vi "Teleop.vi"(10 "Match Info":T1={"Autonomous Elapsed Seconds"=0.0, "TeleOp Elapsed Seconds"=0.0, "Disabled Elapsed Seconds"=0.0, "Visited Autonomous"=FALSE, "Visited TeleOp"=FALSE, "Visited Disabled"=FALSE, "Autonomous Settings"={"Autonomous Style"=enum."Independent", "VI Refnum"=refnum}}, 11 "Call Context":T2) -> ()   [LabVIEW 2015]
doc: "This VI is called for each TeleOp packet received from the DS where the robot is not disabled. It is often used to read from the joysticks and update I/O or to update setpoints for timed control loops. It should complete and return within 20 milliseconds or it may miss DS packets."
uses:
  <vilib>/Rock Robotics/WPI/DriverStation/WPI_DriverStationDerivedRobotMode.ctl
  <vilib>/Rock Robotics/WPI/DriverStation/WPI_DriverStationMatch Info.ctl
  <vilib>/Rock Robotics/WPI/Utilities/WPI_GetSetVariantRefNum.vi
  Robot Global Data.vi
  <vilib>/Rock Robotics/Network Tables/SD Write Number.vi
  <vilib>/Rock Robotics/WPI/Solenoid/Deprecated/WPI_SolenoidSetBool.vi
  <vilib>/Rock Robotics/Network Tables/NT Write Number.vi
  <vilib>/Rock Robotics/Network Tables/NT Write Boolean.vi
  Z navX/navX Library v2/navX Library v2.lvlib
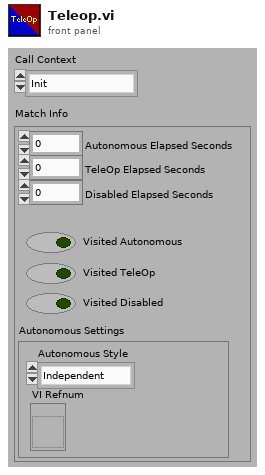
[diagram p1: front panel]
types:
  T1 = typedef "WPI_DriverStationMatch Info.ctl" = cluster{"Autonomous Elapsed Seconds":dbl, "TeleOp Elapsed Seconds":dbl, "Disabled Elapsed Seconds":dbl, "Visited Autonomous":bool, "Visited TeleOp":bool, "Visited Disabled":bool, "Autonomous Settings":cluster{"Autonomous Style":enum16{"Iterative", "Independent"}, "VI Refnum":refnum<vi>}}
  T2 = typedef "WPI_DriverStationDerivedRobotMode.ctl" = enum16{"Init", "Execute", "Stop"}
  T3 = enum16{"No Override", "Override to Coast", "Override to Brake"}
  T4 = typedef "WPI_JoystickDevRef.ctl" = cluster{"Device":T5}
  T5 = typedef "WPI_JoystickDeviceEnum.ctl" = enum16{"USB 0", "USB 1", "USB 2", "USB 3", "USB 4", "USB 5"}
  T6 = cluster{"Axes[0]":dbl, "Axes[1]":dbl, "Axes[2]":dbl, "Axes[3]":dbl, "Axes[4]":dbl, "Axes[5]":dbl, "Axes[6]":dbl, "Axes[7]":dbl, "Axes[8]":dbl}
  T7 = cluster{"Buttons[0]":bool, "Buttons[1]":bool, "Buttons[2]":bool, "Buttons[3]":bool, "Buttons[4]":bool, "Buttons[5]":bool, "Buttons[6]":bool, "Buttons[7]":bool, "Buttons[8]":bool}
  T8 = typedef "navX Library v2.lvlib/Z900_navX_DeviceTypeDef.ctl" = cluster{"Interface":cluster{"Protocol":T9, "Update Rate (4Hz-60Hz)":u8, "navX Open TypeDef":variant}, "Notify Packet":refnum<notifier>, "Loop VI Refnum":refnum<vi>, "Ready to Close Occurrence Refnum":refnum<k4>}
  T9 = typedef "navX Library v2.lvlib/Z900_navX_ProtocolTypeDef.ctl" = enum16{"SERIAL", "I2C", "SPI"}
  T10 = cluster{"Yaw":dbl, "Roll":dbl, "Pitch":dbl, "Heading":dbl, "Fused Heading":dbl}
  T11 = cluster{"LinearAcceleration X":dbl, "LinearAcceleration Y":dbl, "LinearAcceleration Z":dbl}
  T12 = cluster{"Velocity X":dbl, "Velocity Y":dbl, "Velocity Z":dbl, "Displacement X":dbl, "Displacement Y":dbl, "Displacement Z":dbl}
  T13 = typedef "WPI_MotorControlDeviceRef.ctl" = cluster{"DeviceStatus":errorcluster, "Type":T14, "PWM":cluster{"PWM Channel":T15, "DeadBand":T16}, "CAN":cluster{"Device Number":u8, "Control Mode":T17, "Semaphore":T18, "Max Vout":dbl, "TalonSRX Control Mode":T19}, "Invert":bool}
  T14 = typedef "WPI_MotorControlType.ctl" = enum16{"PWM", "CAN", "CANTalonSRX"}
  T15 = typedef "FPGA_DIOPWMChannel.ctl" = enum8{"PWM 0", "PWM 1", "PWM 2", "PWM 3", "PWM 4", "PWM 5", "PWM 6", "PWM 7", "PWM 8", "PWM 9", "PWM MXP 0", "PWM MXP 1", "PWM MXP 2", "PWM MXP 3", "PWM MXP 4", "PWM MXP 5", "PWM MXP 6", "PWM MXP 7", "PWM MXP 8", "PWM MXP 9", "Invalid"}
  T16 = typedef "WPI_PWMDeadband.ctl" = cluster{"Name":string, "maxPositivePwm":i32, "minPositivePwm":i32, "centerPwm":i32, "maxNegativePwm":i32, "minNegativePwm":i32, "angularRange":u16}
  T17 = typedef "WPI_CANJaguar_ControlMode.ctl" = enum8{"Percent VBus", "Current", "Speed", "Position", "Voltage"}
  T18 = typedef "Semaphore RefNum" = refnum<k1>
  T19 = typedef "WPI_CANTalonSRX_APIControlMode.ctl" = enum8{"Percent VBus", "Speed", "Position", "Slave", "Unchanged / Invalid", "Voltage Compensation", "Current", "Motion Profile"}
  T20 = typedef "WPI_SolenoidDevRef.ctl" = cluster{"DevStatus":errorcluster, "Pneumatics Control Module":u8, "Forward Solenoid Channel":T21, "Reverse Solenoid Channel":T21}
  T21 = typedef "WPI_SolenoidChannel.ctl" = enum8{"Solenoid 0", "Solenoid 1", "Solenoid 2", "Solenoid 3", "Solenoid 4", "Solenoid 5", "Solenoid 6", "Solenoid 7", "Invalid"}
  T22 = typedef "WPI_CANTalonSRX_GlobalStatus.ctl" = cluster{"Applied Throttle":dbl, "Module Enabled":bool, "CAN Error":errorcluster, "Closed Loop Error":dbl, "Forward Limit Switch Closed":bool, "Reverse Limit Switch Closed":bool, "Sensor Position":dbl, "Sensor Velocity":dbl, "Current":dbl, "Sticky Fault - Over Temp":bool, "Sticky Fault - Under Voltage":bool, "Sticky Fault - Forward Limit":bool, "Sticky Fault - Reverse Limit":bool, "Sticky Fault - Forward Soft Limit":bool, "Sticky Fault - Reverse Soft Limit":bool, "Brake is Enabled":bool, "Encoder Position":dbl, "Encoder Velocity":dbl, "Encoder Index Count":dbl, "Encoder A Pin State":bool, "Encoder B Pin State":bool, "Encoder Index Pin State":bool, "Analog In":dbl, "Analog In Velocity":dbl, "Temperature (C)":dbl, "Battery Voltage":dbl, "Control 5 Is Supported":bool, "Current Profile Slot Select":dbl, "Pos Div 8":bool, "Vel Div 4":bool, "Pulse Width Position":i32, "Pulse Width Velocity":i32, "Pulse Width Rise To Rise (us)":i32, "Pulse Width Rise To Fall (us)":i32, "Mot Prof Active Is Under Run":bool, "Mot Prof Active Has Under Run":bool, "Mot Prof Active Is Last":bool, "Mot Prof Active Velocity Only":bool, "Mot Prof Active Is Valid":bool, "Mot Prof Buffer Is Full":bool, "Mot Prof Active Profile Slot Select":i32, "Mot Prof NextID":i32, "Mot Prof Count":i32, "Mot Prof Active Velocity":dbl, "Mot Prof Active Position":dbl, "Mot Prof Output Enable":i32}
  T23 = typedef "WPI_RobotDriveDevRef.ctl" = cluster{"DevStatus":errorcluster, "Motors[]":T13[], "Square Inputs":bool, "Max Output":dbl}
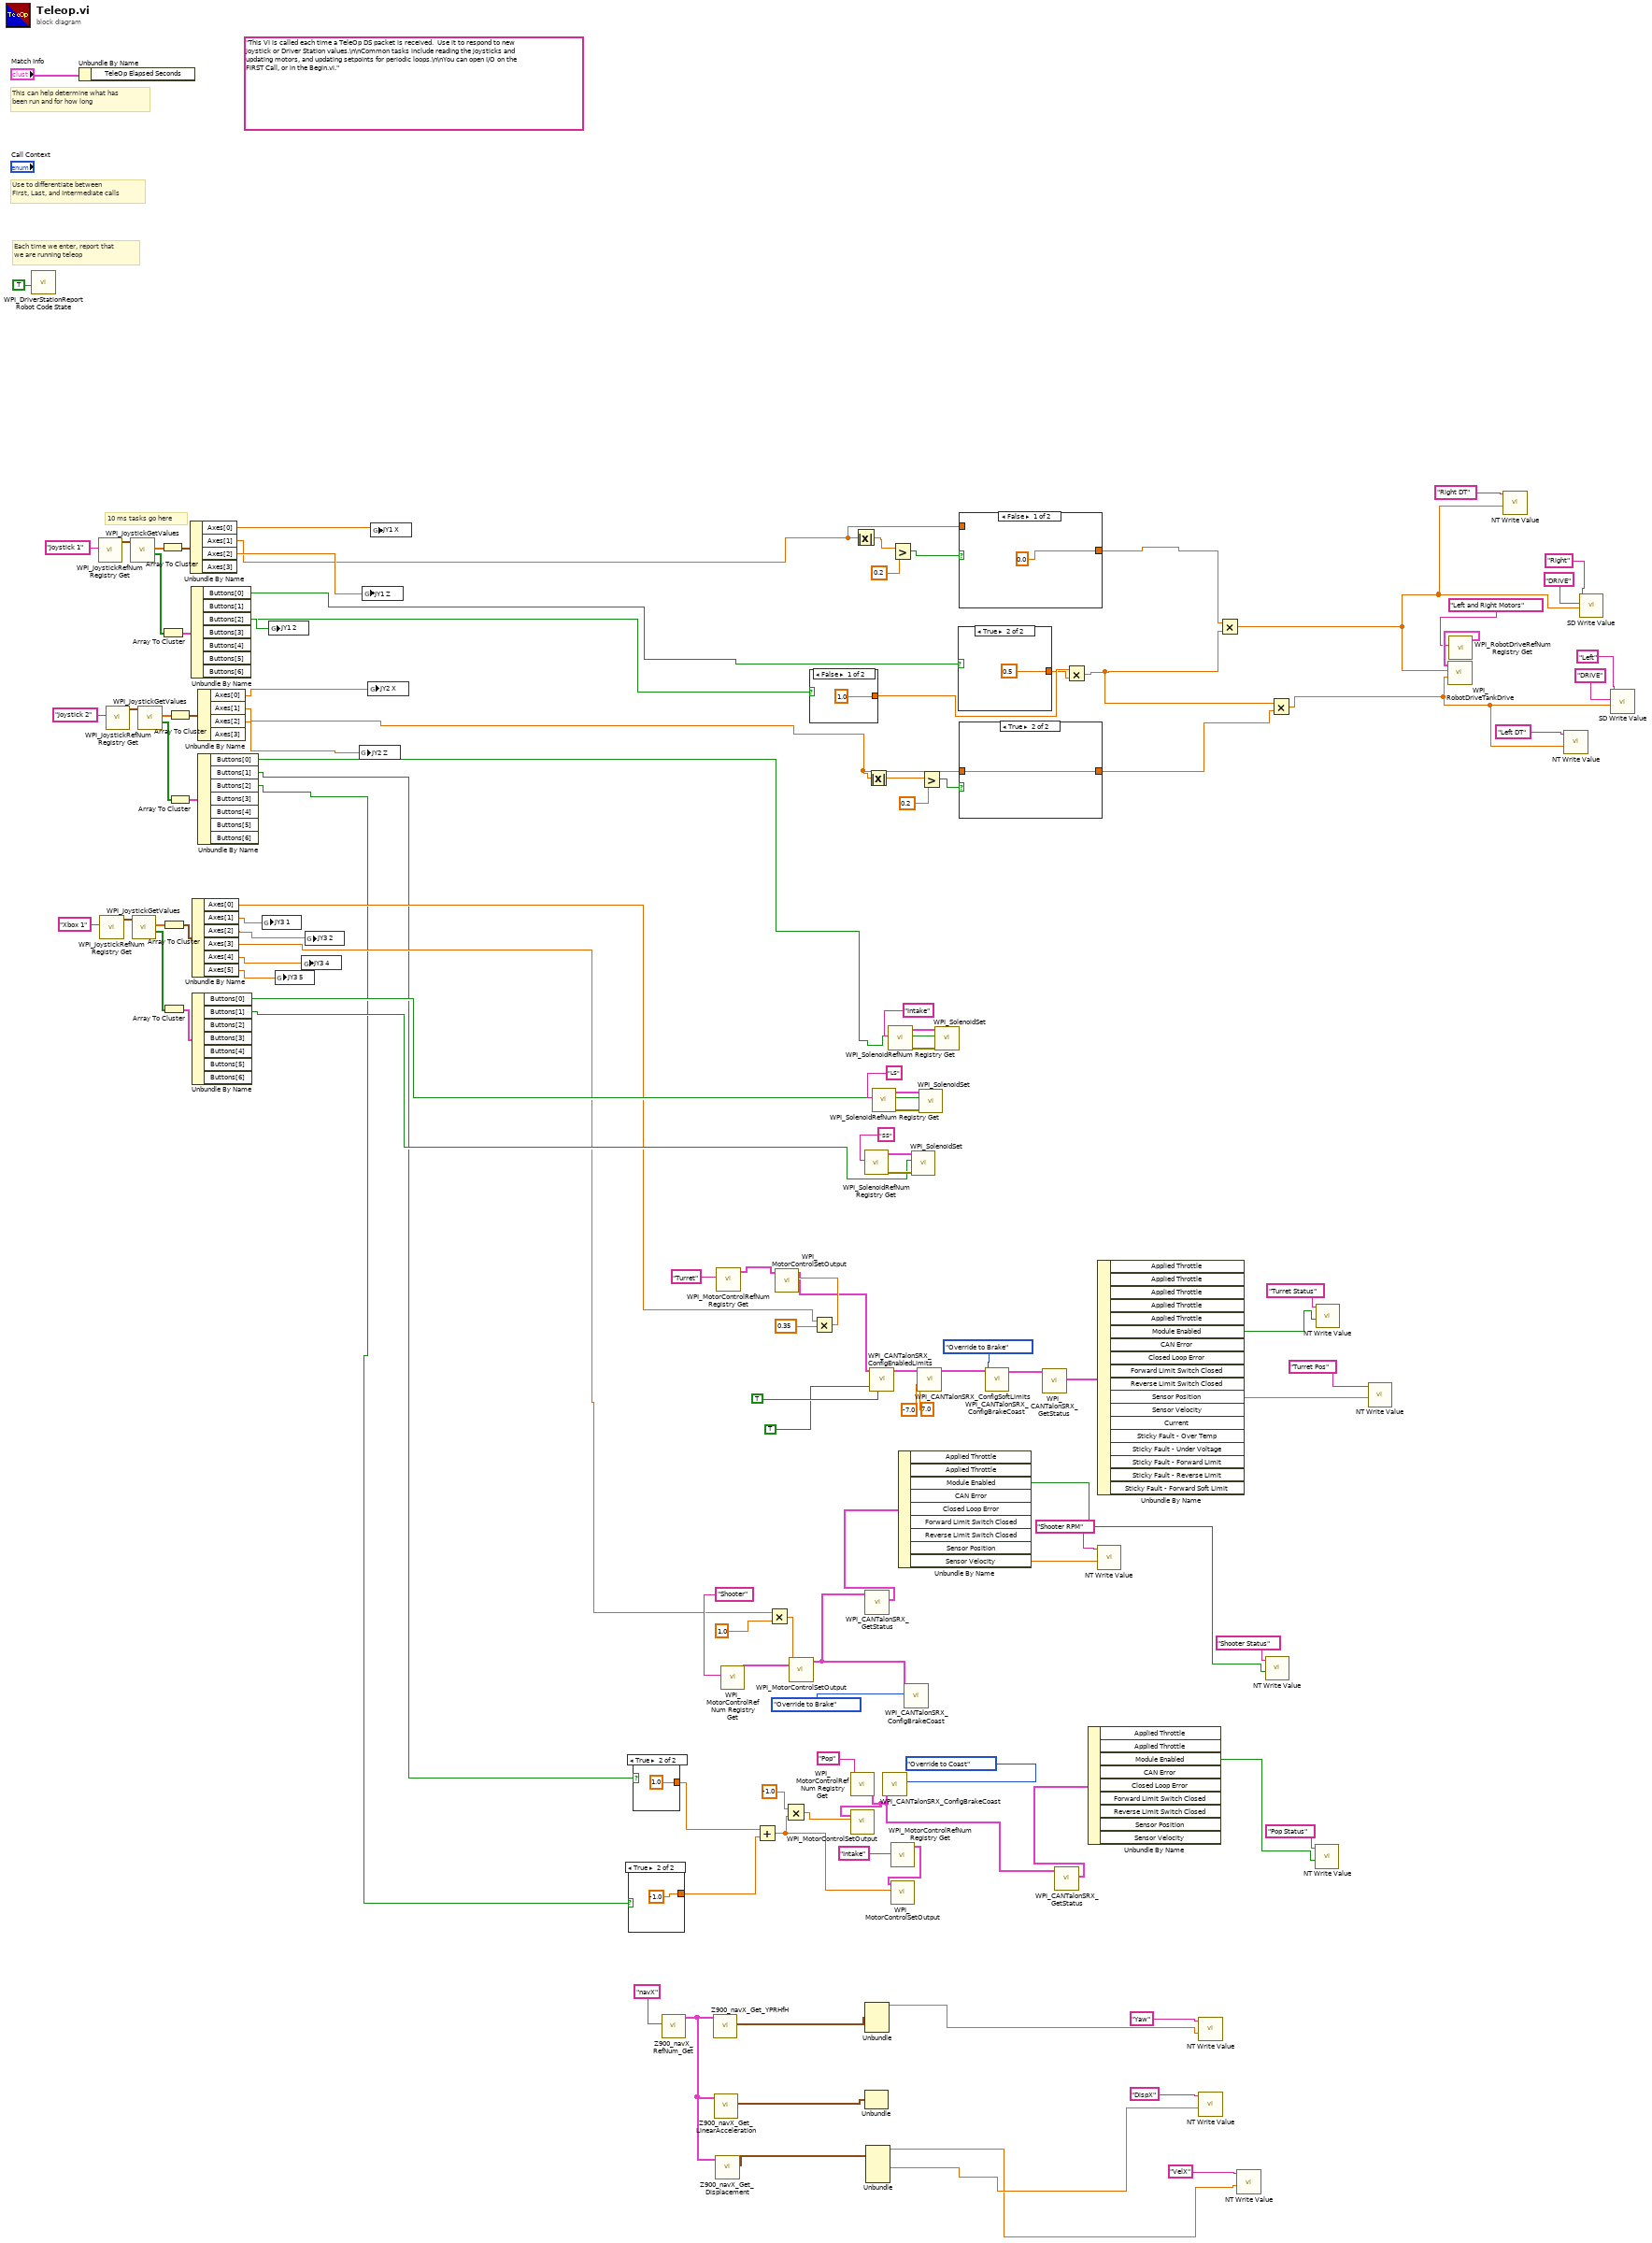
[diagram p0: block diagram]
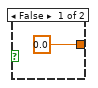
[diagram p2: hidden frame]
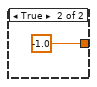
[diagram p3: hidden frame]
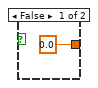
[diagram p4: hidden frame]
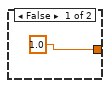
[diagram p5: hidden frame]
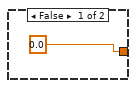
[diagram p6: hidden frame]
diagram:
  (unwired) "This VI is called each time a TeleOp DS packet is received.  Use it to respond to new joystick or Driver Station values.\n\nCommon tasks include reading the joysticks and updating motors, and updating setpoints for periodic loops.\n\nYou can open I/O on the FIRST Call, or in the Begin.vi."
  # "10 ms tasks go here"
  # "Each time we enter, report that\nwe are running teleop"
  # "Use to differentiate between\nFirst, Last, and Intermediate calls"
  # "This can help determine what has\nbeen run and for how long"
  n1 = call <vilib>:"WPI_DriverStationReport Robot Code State.vi"("TeleOp"=TRUE ("Autonomous")) -> ()  [unwired: 10 in, 1 out]
  n2 = Unbundle By Name("Match Info") -> ()  [unwired: 1 out]
  n3 = call <vilib>:"WPI_JoystickRefNum Registry Get.vi"("refnum name"="Joystick 1") -> ("JoystickDevRef"=w77:T4)  [unwired: 1 in, 9 out]
  n4 = call <vilib>:"WPI_JoystickRefNum Registry Get.vi"("refnum name"="Xbox 1") -> ("JoystickDevRef"=w65:T4)  [unwired: 1 in, 9 out]
  n5 = call <vilib>:"WPI_JoystickRefNum Registry Get.vi"("refnum name"="Joystick 2") -> ("JoystickDevRef"=w71:T4)  [unwired: 1 in, 9 out]
  n6 = call <vilib>:"WPI_JoystickGetValues.vi"("JoystickDevRef"=w77) -> ("Buttons"=w75:bool[], "Axes"=w74:dbl[])  [unwired: 6 in, 3 out]
  n7 = call <vilib>:"WPI_JoystickGetValues.vi"("JoystickDevRef"=w65) -> ("Buttons"=w63:bool[], "Axes"=w62:dbl[])  [unwired: 6 in, 3 out]
  n8 = call <vilib>:"WPI_JoystickGetValues.vi"("JoystickDevRef"=w71) -> ("Buttons"=w69:bool[], "Axes"=w68:dbl[])  [unwired: 6 in, 3 out]
  n9 = Array To Cluster(array=w74) -> (cluster=w76:T6)
  n10 = Array To Cluster(array=w75) -> (cluster=w73:T7)
  n11 = Array To Cluster(array=w62) -> (cluster=w64:T6)
  n12 = Array To Cluster(array=w63) -> (cluster=w61:T7)
  n13 = Array To Cluster(array=w68) -> (cluster=w70:T6)
  n14 = Array To Cluster(array=w69) -> (cluster=w67:T7)
  n15 = Unbundle By Name(w76) -> ("Axes[0]"=w59:dbl, "Axes[1]"=w49:dbl, "Axes[2]"=w58:dbl)  [unwired: 1 out]
  n16 = Unbundle By Name(w73) -> ("Buttons[0]"=w51:bool, "Buttons[1]"=w50:bool, "Buttons[2]"=w52:bool)  [unwired: 4 out]
  n17 = Unbundle By Name(w64) -> ("Axes[0]"=w31:dbl, "Axes[1]"=w55:dbl, "Axes[2]"=w53:dbl, "Axes[3]"=w40:dbl, "Axes[4]"=w54:dbl, "Axes[5]"=w60:dbl)
  n18 = Unbundle By Name(w61) -> ("Buttons[0]"=w46:bool, "Buttons[1]"=w45:bool)  [unwired: 5 out]
  n19 = Unbundle By Name(w70) -> ("Axes[0]"=w57:dbl, "Axes[1]"=w48:dbl, "Axes[2]"=w56:dbl)  [unwired: 1 out]
  n20 = Unbundle By Name(w67) -> ("Buttons[0]"=w47:bool, "Buttons[1]"=w24:bool, "Buttons[2]"=w23:bool)  [unwired: 4 out]
  n21 = global write "Robot Global Data.vi" "JY3 1"(w55) -> ()
  n22 = global write "Robot Global Data.vi" "JY1 2"(w52) -> ()
  n23 = global write "Robot Global Data.vi" "JY3 5"(w60) -> ()
  n24 = global write "Robot Global Data.vi" "JY3 4"(w54) -> ()
  n25 = global write "Robot Global Data.vi" "JY3 2"(w53) -> ()
  n26 = global write "Robot Global Data.vi" "JY2 Z"(w56) -> ()
  n27 = global write "Robot Global Data.vi" "JY1 Z"(w58) -> ()
  n28 = global write "Robot Global Data.vi" "JY2 X"(w57) -> ()
  n29 = global write "Robot Global Data.vi" "JY1 X"(w59) -> ()
  n30 = case shown="True" w23 {
    tunnel: [0.0 -1.0] -> w90
    frame False {
    }
    frame True {
    }
  }
  n31 = case shown="True" w24 {
    tunnel: [0.0 1.0] -> w91
    frame False {
    }
    frame True {
    }
  }
  n32 = call "Z900_navX_RefNum_Get.vi"("refnum name"="navX") -> ("navX Device"=w43:T8)  [unwired: 9 in, 1 out]
  n33 = call "Z900_navX_Get_YPRHfH.vi"("navX Device"=w43) -> ("YRPHfH"=w44:T10)  [unwired: 7 in, 3 out]
  n34 = call "Z900_navX_Get_LinearAcceleration.vi"("navX Device"=w43) -> ("Linear Acceleration"=w42:T11)  [unwired: 7 in, 3 out]
  n35 = call "Z900_navX_Get_Displacement.vi"("navX Device"=w43) -> ("Displacement"=w41:T12)  [unwired: 7 in, 3 out]
  n36 = call <vilib>:"WPI_MotorControlRefNum Registry Get.vi"("refnum name"="Turret") -> ("MotorControlDevRef"=w30:T13)  [unwired: 9 in, 1 out]
  n37 = call <vilib>:"WPI_MotorControlRefNum Registry Get.vi"("refnum name"="Shooter") -> ("MotorControlDevRef"=w86:T13)  [unwired: 9 in, 1 out]
  n38 = Add(x=w91, y=w90) -> (x+y=w84:dbl)
  n39 = Multiply(x=w40, y=1.0) -> (x*y=w89:dbl)
  n40 = Multiply(x=-1.0, y=w84) -> (x*y=w85:dbl)
  n41 = call <vilib>:"WPI_MotorControlSetOutput.vi"("Output"=w89, "MotorControlDevRef"=w86) -> ("MotorControlDevRef"=w81:T13)  [unwired: 7 in, 2 out]
  n42 = case shown="False" w50 {
    tunnel: [1.0 -1.0] -> w96
    frame False {
    }
    frame True {
    }
  }
  n43 = Multiply(x=w31, y=0.35) -> (x*y=w38:dbl)
  n44 = call <vilib>:"WPI_MotorControlSetOutput.vi"("Output"=w38, "MotorControlDevRef"=w30) -> ("MotorControlDevRef"=w29:T13)  [unwired: 7 in, 2 out]
  n45 = call <vilib>:"WPI_MotorControlRefNum Registry Get.vi"("refnum name"="Pop") -> ("MotorControlDevRef"=w3:T13)  [unwired: 9 in, 1 out]
  n46 = call <vilib>:"WPI_MotorControlSetOutput.vi"("Output"=w85, "MotorControlDevRef"=w3) -> ()  [unwired: 7 in, 3 out]
  n47 = Absolute Value(x=w49) -> (abs(x)=w117:dbl)
  n48 = call <vilib>:"WPI_SolenoidRefNum Registry Get.vi"("refnum name"="SS") -> ("error out"=w103:errorcluster, "SolenoidDevRef"=w104:T20)  [unwired: 9 in]
  n49 = Unbundle(w42) -> ()  [unwired: 3 out]
  n50 = call <vilib>:"WPI_CANTalonSRX_GetStatus.vi"("CAN Talon SRX Ref"=w81) -> ("Talon SRX Status"=w87:T22)  [unwired: 8 in, 2 out]
  n51 = Unbundle(w44) -> ("Yaw"=w10:dbl)  [unwired: 4 out]
  n52 = Unbundle(w41) -> ("Velocity X"=w8:dbl, "Displacement X"=w12:dbl)  [unwired: 4 out]
  n53 = Absolute Value(x=w48) -> (abs(x)=w116:dbl)
  n54 = call <vilib>:"WPI_CANTalonSRX_ConfigEnabledLimits.vi"("CAN Talon SRX Ref"=w29, "Forward Soft Limit Enable"=TRUE, "Reverse Soft Limit Enable"=TRUE) -> ("CAN Talon SRX Ref"=w28:T13)  [unwired: 11 in, 1 out]
  n55 = call <vilib>:"WPI_SolenoidRefNum Registry Get.vi"("refnum name"="LS") -> ("error out"=w106:errorcluster, "SolenoidDevRef"=w107:T20)  [unwired: 9 in]
  n56 = call <vilib>:"WPI_CANTalonSRX_ConfigBrakeCoast.vi"("Brake / Coast Mode"=T3."Override to Coast", "CAN Talon SRX Ref"=w3) -> ()  [unwired: 8 in, 2 out]
  n57 = call <vilib>:"WPI_SolenoidRefNum Registry Get.vi"("refnum name"="Intake") -> ("error out"=w100:errorcluster, "SolenoidDevRef"=w101:T20)  [unwired: 9 in]
  n58 = Greater?(x=w117, y=0.2) -> (0:w121:bool)
  n59 = call <vilib>:"WPI_MotorControlRefNum Registry Get.vi"("refnum name"="Intake") -> ("MotorControlDevRef"=w92:T13)  [unwired: 9 in, 1 out]
  n60 = call <vilib>:"WPI_MotorControlSetOutput.vi"("Output"=w84, "MotorControlDevRef"=w92) -> ()  [unwired: 7 in, 3 out]
  n61 = Unbundle By Name(w87) -> ("Module Enabled"=w6:bool, "Sensor Velocity"=w18:dbl)  [unwired: 7 out]
  n62 = call <vilib>:"WPI_CANTalonSRX_ConfigBrakeCoast.vi"("Brake / Coast Mode"=T3."Override to Brake", "CAN Talon SRX Ref"=w81) -> ()  [unwired: 8 in, 2 out]
  n63 = call-poly <vilib>:"WPI_SolenoidSet.vi"("error in (no error)"=w103, "Value"=w45, "SolenoidDevRef"=w104) -> ()  [unwired: 9 out]
  n64 = call <vilib>:"WPI_CANTalonSRX_ConfigSoftLimits.vi"("CAN Talon SRX Ref"=w28, "Forward Limit Position"=7.0, "Reverse Limit Position"=-7.0) -> ("CAN Talon SRX Ref"=w27:T13)  [unwired: 11 in, 1 out]
  n65 = call-poly <vilib>:"WPI_SolenoidSet.vi"("error in (no error)"=w106, "Value"=w46, "SolenoidDevRef"=w107) -> ()  [unwired: 9 out]
  n66 = Greater?(x=w116, y=0.2) -> (0:w119:bool)
  n67 = call-poly <vilib>:"WPI_SolenoidSet.vi"("error in (no error)"=w100, "Value"=w47, "SolenoidDevRef"=w101) -> ()  [unwired: 9 out]
  n68 = case shown="True" w51 {
    tunnel: [1.0 0.5] -> w94
    frame False {
    }
    frame True {
    }
  }
  n69 = case shown="False" w121 {
    tunnel: [0.0 w133] -> w110
    tunnel: w49 -> [_ w133]
    frame False {
    }
    frame True {
    }
  }
  n70 = case shown="True" w119 {
    tunnel: [0.0 w135] -> w111
    tunnel: w48 -> [_ _]
    tunnel: w48 -> [_ w135]
    frame False {
    }
    frame True {
    }
  }
  n71 = call <vilib>:"WPI_CANTalonSRX_ConfigBrakeCoast.vi"("Brake / Coast Mode"=T3."Override to Brake", "CAN Talon SRX Ref"=w27) -> ("CAN Talon SRX Ref"=w26:T13)  [unwired: 8 in, 1 out]
  n72 = call <vilib>:"WPI_CANTalonSRX_GetStatus.vi"("CAN Talon SRX Ref"=w26) -> ("Talon SRX Status"=w25:T22)  [unwired: 8 in, 2 out]
  n73 = call <vilib>:"WPI_CANTalonSRX_GetStatus.vi"("CAN Talon SRX Ref"=w3) -> ("Talon SRX Status"=w4:T22)  [unwired: 8 in, 2 out]
  n74 = Multiply(x=w96, y=w94) -> (x*y=w95:dbl)
  n75 = Unbundle By Name(w4) -> ("Module Enabled"=w2:bool)  [unwired: 8 out]
  n76 = call-poly <vilib>:"NT Write Value.vi"("Numeric"=w18, "Name"="Shooter RPM") -> ()  [unwired: 9 in, 1 out]
  n77 = Unbundle By Name(w25) -> ("Module Enabled"=w19:bool, "Sensor Position"=w22:dbl)  [unwired: 16 out]
  n78 = call-poly <vilib>:"NT Write Value.vi"("Numeric"=w10, "Name"="Yaw") -> ()  [unwired: 9 in, 1 out]
  n79 = call-poly <vilib>:"NT Write Value.vi"("Numeric"=w12, "Name"="DispX") -> ()  [unwired: 9 in, 1 out]
  n80 = Multiply(x=w110, y=w95) -> (x*y=w14:dbl)
  n81 = call-poly <vilib>:"NT Write Value.vi"("Numeric"=w8, "Name"="VelX") -> ()  [unwired: 9 in, 1 out]
  n82 = call-poly <vilib>:"NT Write Value.vi"("Boolean"=w6, "Name"="Shooter Status") -> ()  [unwired: 9 in, 1 out]
  n83 = Multiply(x=w95, y=w111) -> (x*y=w16:dbl)
  n84 = call-poly <vilib>:"NT Write Value.vi"("Boolean"=w2, "Name"="Pop Status") -> ()  [unwired: 9 in, 1 out]
  n85 = call-poly <vilib>:"NT Write Value.vi"("Boolean"=w19, "Name"="Turret Status") -> ()  [unwired: 9 in, 1 out]
  n86 = call-poly <vilib>:"NT Write Value.vi"("Numeric"=w22, "Name"="Turret Pos") -> ()  [unwired: 9 in, 1 out]
  n87 = call <vilib>:"WPI_RobotDriveRefNum Registry Get.vi"("refnum name"="Left and Right Motors") -> ("RobotDriveDevRef"=w109:T23)  [unwired: 9 in, 1 out]
  n88 = call <vilib>:"WPI_RobotDriveTankDrive.vi"("Right axis value"=w16, "Left axis value"=w14, "RobotDriveDevRef"=w109) -> ()  [unwired: 6 in, 3 out]
  n89 = call-poly <vilib>:"NT Write Value.vi"("Numeric"=w14, "Name"="Right DT") -> ()  [unwired: 9 in, 1 out]
  n90 = call-poly <vilib>:"NT Write Value.vi"("Numeric"=w16, "Name"="Left DT") -> ()  [unwired: 9 in, 1 out]
  n91 = call-poly <vilib>:"SD Write Value.vi"("Numeric"=w14, "Table Prefix"="DRIVE", "Name"="Right") -> ()  [unwired: 7 in, 2 out]
  n92 = call-poly <vilib>:"SD Write Value.vi"("Numeric"=w16, "Table Prefix"="DRIVE", "Name"="Left") -> ()  [unwired: 7 in, 2 out]
